vi "Define.vi"(11 "Integer Definition":T1) -> (3 "Integer out":refnum<class "Integer.lvclass">)   [LabVIEW 2022 SP3, in "Conditum.lvlib" / "Columns.lvlib" / "Integer.lvclass"]
uses:
  Integer.lvclass
  C:/dev/lv/illuminated-g/lv-conditum/Conditum/Columns/Type/Type.lvclass
  Integer Definition.ctl
  Type/Definition.ctl
  Attributes.ctl
  Definition.ctl
  Type/Type.lvclass/Type.ctl
  Integer.lvclass/Integer.ctl
  Type/Type.lvclass
  LabVIEW Type.ctl
  Conditum.lvlib
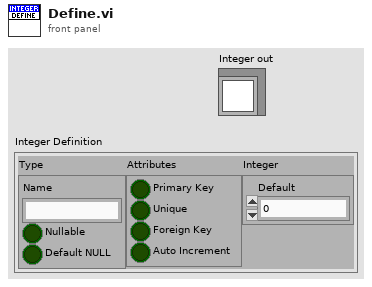
[diagram p1: front panel]
types:
  T1 = typedef "Conditum.lvlib/Columns.lvlib/Integer.lvclass/Integer Definition.ctl" = cluster{"Type":T2, "Attributes":T3, "Integer":T4}
  T2 = typedef "Conditum.lvlib/Columns.lvlib/Type.lvclass/Definition.ctl" = cluster{"Name":string, "Nullable":bool, "Default NULL":bool}
  T3 = typedef "Conditum.lvlib/Attributes.ctl" = cluster{"Primary Key":bool, "Unique":bool, "Foreign Key":bool, "Auto Increment":bool}
  T4 = typedef "Conditum.lvlib/Columns.lvlib/Integer.lvclass/Definition.ctl" = cluster{"Default":i64}
  T5 = typedef "Conditum.lvlib/LabVIEW Type.ctl" = enum16{"None", "ID", "Boolean", "Integer", "Double", "Timestamp", "String", "Text", "Entity"}
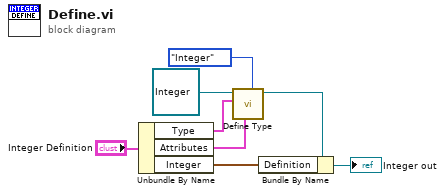
[diagram p0: block diagram]
diagram:
  n1 = Unbundle By Name("Integer Definition") -> ("Type"=w6:T2, "Attributes"=w2:T3, "Integer"=w5:T4)
  n2 = call "Define Type.vi"("Type"=LabVIEW_Type."Integer", "Attributes"=w2, "Definition"=w6, "Type in"=refnum<class "Integer.lvclass"> refnum ("Integer out")) -> ("Type out"=w4:refnum<class "Integer.lvclass">)  [unwired: 7 in]
  n3 = Bundle By Name(cluster=w4, "Definition"=w5) -> (→"Integer out":refnum<class "Integer.lvclass">)
